vi "Read Headers.vi"(8 "error in (no error)":errorcluster, 10 "Header Names":string[](array[string]), 11 "Linked List Definition in":refnum<class "Linked List Definition.lvclass">) -> (0 "error out":errorcluster, 1 "Header Values":string[](array[string]), 2 "Header Names":string[](array[string]), 3 "Linked List Definition out":refnum<class "Linked List Definition.lvclass">, 4 "Found?":bool)   [LabVIEW 2020, in "Linked Lists.lvlib" / "Linked List Definition.lvclass"]
uses:
  <vilib>/gpm_packages/@cs/linked-list/Source/Linked List/Linked List Definition/Linked List Definition.lvclass
  <vilib>/gpm_packages/@cs/linked-list/Source/Linked List/Linked List Definition/Linked List Definition.lvclass/Linked List Definition.ctl
  <vilib>/gpm_packages/@cs/linked-list/Source/Linked List/Linked List Header/Linked List Header.lvclass
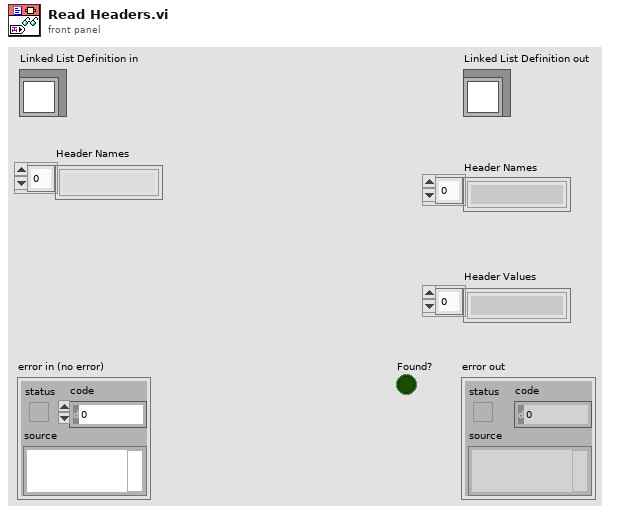
[diagram p1: front panel]
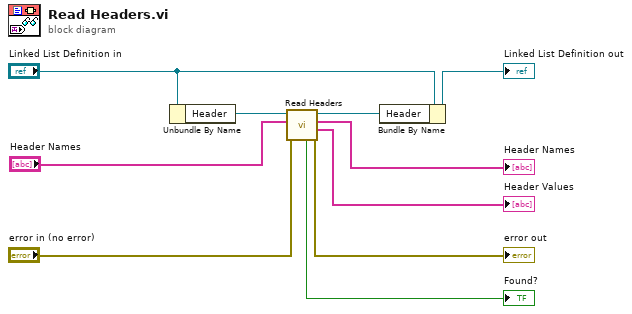
[diagram p0: block diagram]
diagram:
  n1 = Unbundle By Name("Linked List Definition in") -> ("Header"=w10:refnum<class "Linked List Header.lvclass">)
  n2 = call <vilib>:"Read Headers.vi"("error in (no error)"="error in (no error)", "Header Names"="Header Names", "Linked List Header in"=w10) -> ("error out"=→"error out":errorcluster, "Header Values"=→"Header Values":string[], "Header Names"=→"Header Names":string[], "Linked List Header out"=w6:refnum<class "Linked List Header.lvclass">, "Found?"=→"Found?":bool)  [unwired: 4 in]
  n3 = Bundle By Name(cluster="Linked List Definition in", "Header"=w6) -> (→"Linked List Definition out":refnum<class "Linked List Definition.lvclass">)
